vi "PQnfields.vi"(8 "error in (no error)":errorcluster, 10 "res":u64) -> (0 "error out":errorcluster, 1 "PQnFields":i64, 2 "res out":u64)   [LabVIEW 2019, in "libpqlv64.lvlib"]
doc: "Returns the number of columns (fields) in each row of the query result."
uses:
  libpqlv64.lvlib
  libpq.dll
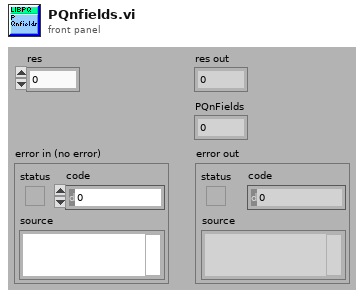
[diagram p1: front panel]
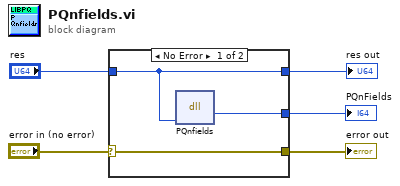
[diagram p0: block diagram]
diagram:
  n1 = case shown="No Error" "error in (no error)" {
    selector: "error in (no error)" -> [w8 w10]
    tunnel: [w8 w10] -> w4
    tunnel: [w7 _] -> w3
    tunnel: "res" -> [w6 w9]
    tunnel: [w6 w9] -> w1
    frame No Error {
      n2 = dll-call lib="libpq.*" fn="PQnfields"("res"=w6) -> ("PQnFields"=w7:i64)  [unwired: 4 in, 2 out]
    }
    frame Error {
    }
  }
  "PQnFields" <- w3
  "error out" <- w4
  "res out" <- w1
